vi "Write Laser Configuration.vi"(8 "error in (no error)":errorcluster, 10 "Laser Configuration":T1[](array[typedef]), 11 "Laser Quantum in":refnum<class "Laser.lvclass">) -> (0 "error out":errorcluster, 3 "Laser Quantum out":refnum<class "Laser.lvclass">)   [LabVIEW 2018, in "Laser.lvlib" / "Laser.lvclass"]
uses:
  Laser.lvclass
  Resources/Type Defs/Laser Configuration.ctl
  Laser.lvclass/Laser.ctl
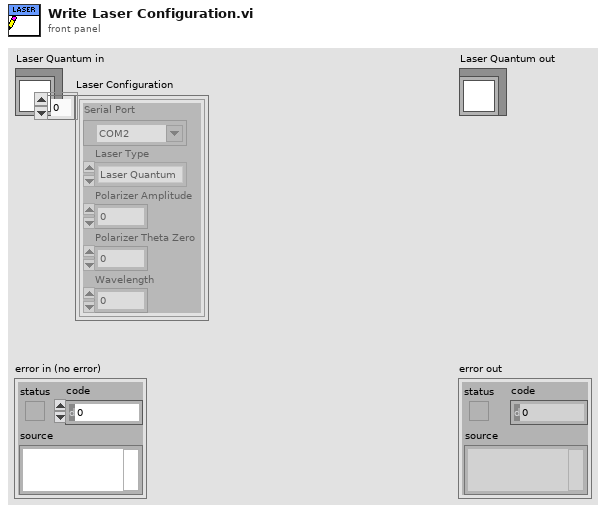
[diagram p1: front panel]
types:
  T1 = typedef "Laser Configuration.ctl" = cluster{"Serial Port":refnum<visa-resource-name>, "Laser Type":enum16{"Disable", "Laser Quantum", "Coherent OBIS", "PRM1-Z8", "Coherent HOPS"}, "Polarizer Amplitude":dbl, "Polarizer Theta Zero":dbl, "Wavelength":u16}
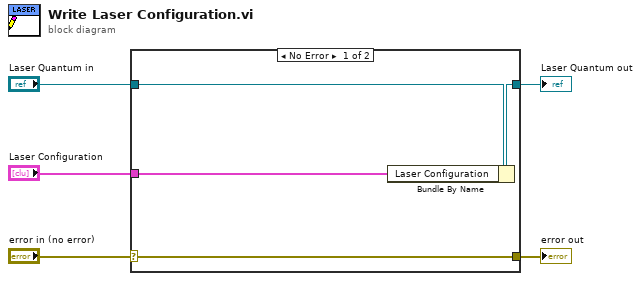
[diagram p0: block diagram]
diagram:
  n1 = case shown="No Error" "error in (no error)" {
    selector: "error in (no error)" -> [w9 w10]
    tunnel: [w9 w10] -> w4
    tunnel: [w7 w11] -> w2
    tunnel: "Laser Quantum in" -> [w8 w11]
    tunnel: "Laser Configuration" -> [w6 _]
    frame No Error {
      n2 = Bundle By Name(cluster=w8, "Laser Configuration"=w6) -> (w7:refnum<class "Laser.lvclass">)
    }
    frame Error {
    }
  }
  "error out" <- w4
  "Laser Quantum out" <- w2
